vi "序列号读取.vi"(8 "Error in":errorcluster caption="Error in (no error)", 11 "MB session in":refnum<class "MB_Master.lvclass">) -> (0 "error out":errorcluster, 2 "序列号":string, 3 "MB session out":refnum<class "MB_Master.lvclass">)   [LabVIEW 2022 SP3, in "斯坦道CODcr.lvlib"]
uses:
  <vilib>/Plasmionique/MB Master/MB_Master/MB_Master.lvclass
  <vilib>/Plasmionique/MB Master/MB Master.lvlib
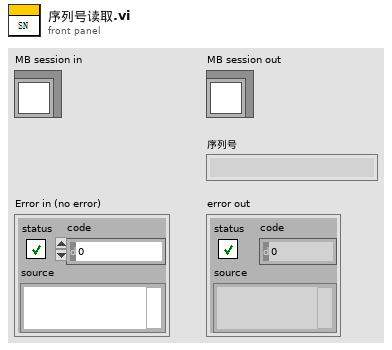
[diagram p1: front panel]
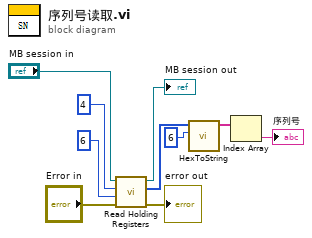
[diagram p0: block diagram]
diagram:
  n1 = call <vilib>:"Read Holding Registers.vi"("error in (no error)"="Error in", "quantity"=u16 6, "starting address"=u16 4, "MB session in"="MB session in") -> ("error out"=→"error out":errorcluster, "Registers"=w4:u16[], "MB session out"=→"MB session out":refnum<class "MB_Master.lvclass">)  [unwired: 5 in]
  n2 = call "HexToString.vi"("字符个数"=6, "数组"=w4) -> ("STRING"=w2:string[])  [unwired: 9 in]
  n3 = Index Array(array=w2) -> (element=→"序列号":string)  [unwired: 1 in]
